vi "Format DescribeInstances_LVXML_ReservationSet.vi"(0 "AWS_EC2 in":refnum<class "AWS_EC2.lvclass">, 1 "xmlDataIn":T18, 3 "error in (no error)":errorcluster) -> (7 "AWS_EC2 out":refnum<class "AWS_EC2.lvclass">, 8 "reservationSet":T1[](array[typedef]), 10 "error IO":errorcluster)   [LabVIEW 2014, in "AWS_EC2.lvlib" / "AWS_EC2.lvclass"]
uses:
  AWS_EC2.lvclass
  lv-xml-parser/r0/trunk/VI Source/EventType.ctl
  EC2 Datatypes/ReservationInfoType.ctl
  EC2 Datatypes/GroupItemType.ctl
  EC2 Datatypes/RunningInstancesItemsType.ctl
  EC2 Datatypes/InstanceStateType.ctl
  EC2 Datatypes/ProductCodeSetItemType.ctl
  EC2 Datatypes/PlacementResponseType.ctl
  EC2 Datatypes/GroupItemTypeSet.ctl
  EC2 Datatypes/StateReasonType.ctl
  EC2 Datatypes/InstanceBlockDeviceMappingResponseItemType.ctl
  EC2 Datatypes/EbsInstanceBlockDeviceMappingResponseType.ctl
  EC2 Datatypes/ResourceTagSetItemType.ctl
  EC2 Datatypes/InstanceNetworkInterfaceSetItemType.ctl
  EC2 Datatypes/InstanceNetworkInterfaceAttachmentType.ctl
  EC2 Datatypes/InstanceNetworkInterfaceAssociationType.ctl
  EC2 Datatypes/InstancePrivateIpAddressesSetItemType.ctl
  EC2 Datatypes/IamInstanceProfileResponseType.ctl
  lv-xml-parser/r0/trunk/VI Source/LV XML Parser.lvlib
  AWS_EC2.lvlib
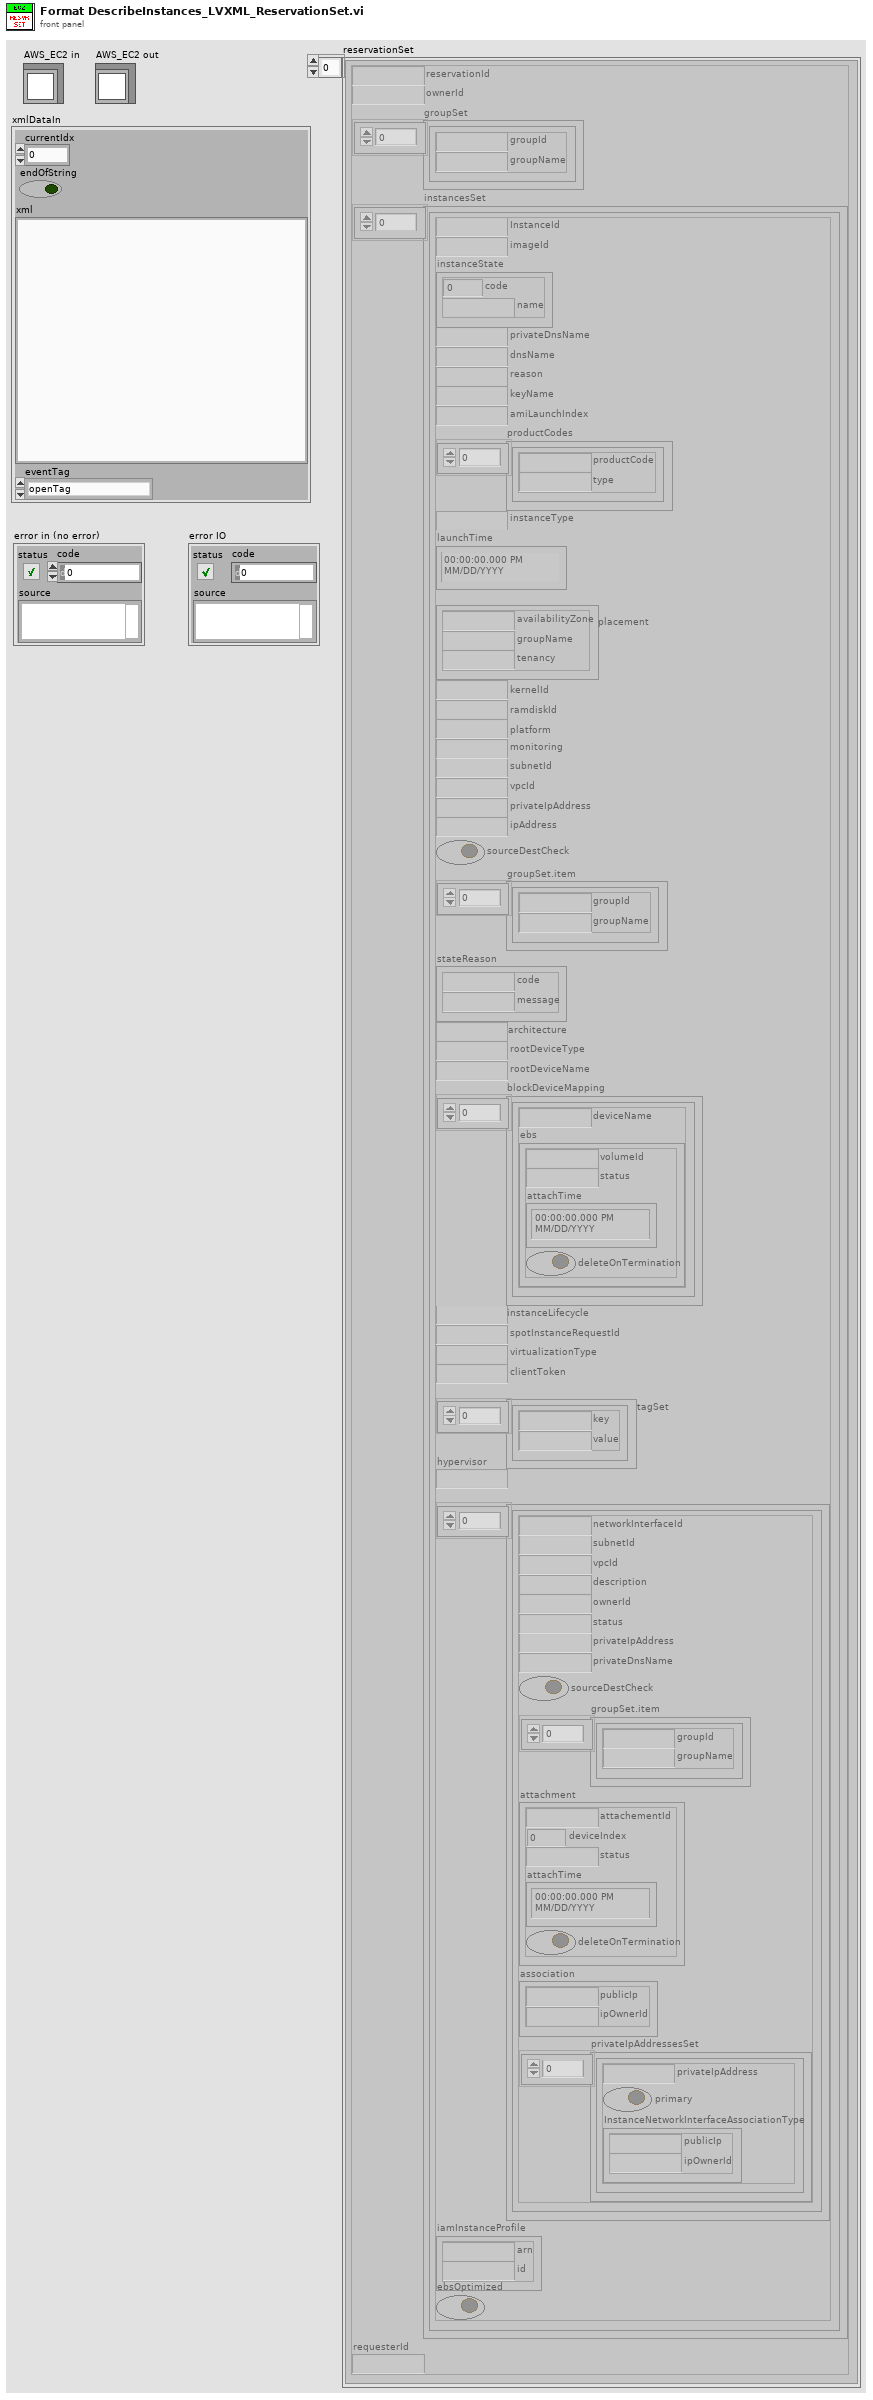
[diagram p1: front panel]
types:
  T1 = typedef "AWS_EC2.lvlib/ReservationInfoType.ctl" = cluster{"reservationId":string, "ownerId":string, "groupSet":T2[], "instancesSet":T3[], "requesterId":string}
  T2 = typedef "AWS_EC2.lvlib/GroupItemType.ctl" = cluster{"groupId":string, "groupName":string}
  T3 = typedef "AWS_EC2.lvlib/RunningInstancesItemsType.ctl" = cluster{"InstanceId":string, "imageId":string, "instanceState":T4, "privateDnsName":string, "dnsName":string, "reason":string, "keyName":string, "amiLaunchIndex":string, "productCodes":T5[], "instanceType":string, "launchTime":timestamp, "placement":T6, "kernelId":string, "ramdiskId":string, "platform":string, "monitoring":string, "subnetId":string, "vpcId":string, "privateIpAddress":string, "ipAddress":string, "sourceDestCheck":bool, "groupSet.item":T7, "stateReason":T8, "architecture":string, "rootDeviceType":string, "rootDeviceName":string, "blockDeviceMapping":T9[], "instanceLifecycle":string, "spotInstanceRequestId":string, "virtualizationType":string, "clientToken":string, "tagSet":T11[], "hypervisor":string, "networkInterfaceSet":T12[], "iamInstanceProfile":T16, "ebsOptimized":bool}
  T4 = typedef "AWS_EC2.lvlib/InstanceStateType.ctl" = cluster{"code":i16, "name":string}
  T5 = typedef "AWS_EC2.lvlib/ProductCodeSetItemType.ctl" = cluster{"productCode":string, "type":string}
  T6 = typedef "AWS_EC2.lvlib/PlacementResponseType.ctl" = cluster{"availabilityZone":string, "groupName":string, "tenancy":string}
  T7 = typedef "AWS_EC2.lvlib/GroupItemTypeSet.ctl" = T2[]
  T8 = typedef "AWS_EC2.lvlib/StateReasonType.ctl" = cluster{"code":string, "message":string}
  T9 = typedef "AWS_EC2.lvlib/InstanceBlockDeviceMappingResponseItemType.ctl" = cluster{"deviceName":string, "ebs":T10}
  T10 = typedef "AWS_EC2.lvlib/EbsInstanceBlockDeviceMappingResponseType.ctl" = cluster{"volumeId":string, "status":string, "attachTime":timestamp, "deleteOnTermination":bool}
  T11 = typedef "AWS_EC2.lvlib/ResourceTagSetItemType.ctl" = cluster{"key":string, "value":string}
  T12 = typedef "AWS_EC2.lvlib/InstanceNetworkInterfaceSetItemType.ctl" = cluster{"networkInterfaceId":string, "subnetId":string, "vpcId":string, "description":string, "ownerId":string, "status":string, "privateIpAddress":string, "privateDnsName":string, "sourceDestCheck":bool, "groupSet.item":T7, "attachment":T13, "association":T14, "privateIpAddressesSet":T15[]}
  T13 = typedef "AWS_EC2.lvlib/InstanceNetworkInterfaceAttachmentType.ctl" = cluster{"attachementId":string, "deviceIndex":i32, "status":string, "attachTime":timestamp, "deleteOnTermination":bool}
  T14 = typedef "AWS_EC2.lvlib/InstanceNetworkInterfaceAssociationType.ctl" = cluster{"publicIp":string, "ipOwnerId":string}
  T15 = typedef "AWS_EC2.lvlib/InstancePrivateIpAddressesSetItemType.ctl" = cluster{"privateIpAddress":string, "primary":bool, "InstanceNetworkInterfaceAssociationType":T14}
  T16 = typedef "AWS_EC2.lvlib/IamInstanceProfileResponseType.ctl" = cluster{"arn":string, "id":string}
  T17 = typedef "LV XML Parser.lvlib/EventType.ctl" = enum16{"openTag", "endOpenTag", "closeTag", "comment", "endComment", "endOfFile", "attribute", "startXml"}
  T18 = cluster{"currentIdx":i32, "endOfString":bool, "xml":string, "eventTag":T17}
  T19 = cluster{"namespaceUri":string, "localName":string}
  T20 = cluster{"Attributes":cluster{"localName":string, "namespaceUri":string, "value":string}[], "localName":string, "namespaceUri":string, "valueXmlData":cluster{"currentIdx":i64, "endOfString":bool, "xml":string, "eventTag":T17}}[]
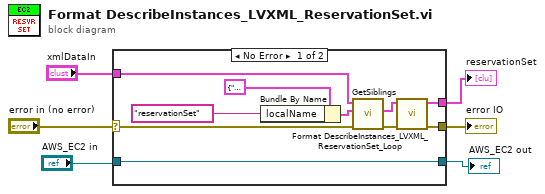
[diagram p0: block diagram]
diagram:
  n1 = case shown="No Error" "error in (no error)" {
    selector: "error in (no error)" -> [w9 w18]
    tunnel: "xmlDataIn" -> [w10 _]
    tunnel: [w11 w18] -> w5
    tunnel: [w8 _] -> w3
    tunnel: "AWS_EC2 in" -> [w7 w17]
    tunnel: [w7 w17] -> w2
    frame No Error {
      n2 = Bundle By Name(cluster=T19 {"namespaceUri"="", "localName"=""} ("limitToTag"), "localName"="reservationSet" ("Tag name")) -> (w14:T19)
      n3 = call "GetSiblings.vi"("error in (no error)"=w9, "limitToTag"=w14, "xmlData"=w10) -> ("error out"=w12:errorcluster, "Siblings"=w13:T20)  [unwired: 7 in]
      n4 = call "Format DescribeInstances_LVXML_ReservationSet_Loop.vi"("error in (no error)"=w12, "Siblings"=w13) -> ("error out"=w11:errorcluster, "reservationSet"=w8:T1[])  [unwired: 8 in]
    }
    frame Error {
    }
  }
  "error IO" <- w5
  "reservationSet" <- w3
  "AWS_EC2 out" <- w2
